vi "write builder settings.vi"(10 "builder settings":T1, 11 "Builder in":refnum<class "Builder.lvclass">) -> (3 "Builder out":refnum<class "Builder.lvclass">)   [LabVIEW 2024, in "Builder.lvclass"]
uses:
  Builder.lvclass
  Builder.lvclass/Builder.ctl
  typedefs/builder settings.ctl
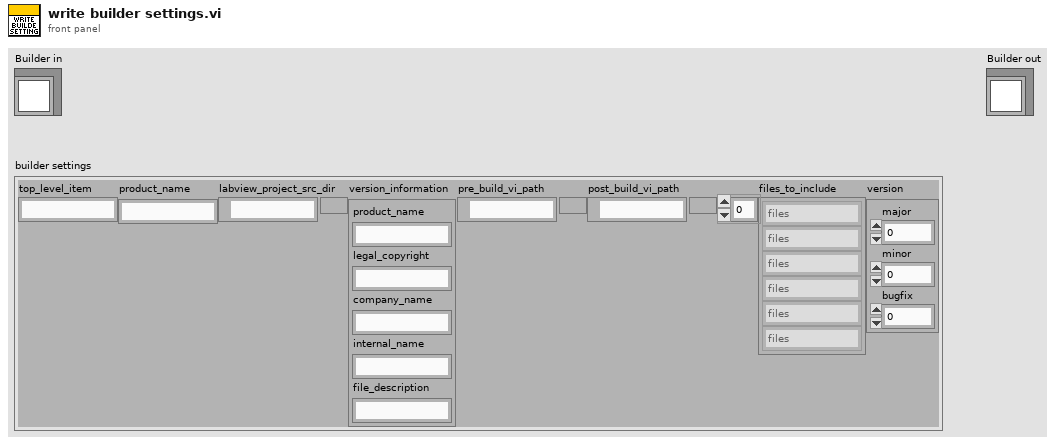
[diagram p1: front panel]
types:
  T1 = typedef "Builder.lvclass/builder settings.ctl" = cluster{"top_level_item":string, "product_name":string, "labview_project_src_dir":path, "version_information":cluster{"product_name":string, "legal_copyright":string, "company_name":string, "internal_name":string, "file_description":string}, "pre_build_vi_path":path, "post_build_vi_path":path, "files_to_include":string[], "version":cluster{"major":u16, "minor":u16, "bugfix":u16}}
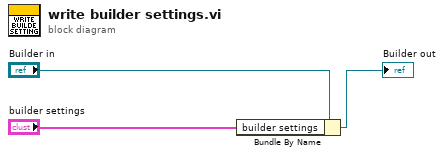
[diagram p0: block diagram]
diagram:
  n1 = Bundle By Name(cluster="Builder in", "builder settings"="builder settings") -> (→"Builder out":refnum<class "Builder.lvclass">)
